vi "CH_LM Config Statistics Histogram Bin Count.vi"(0 "Meter Index":i32, 2 "Number of Bins (7)":i32=7, 5 "error in (no error)":errorcluster, 7 "Timeout / ms (3000)":i32=3000, 8 "Action (query)":bool, 9 "Lock Timeout / ms (1000)":i32=1000) -> (11 "Lock timed out":bool, 14 "Meter Index":i32, 16 "Number of Bins":i32, 19 "error out":errorcluster)   [LabVIEW 2012, in "CH_LM.lvlib"]
doc: "This command will set/query the statistics histogram bin count, which takes effect at the end of the current statistical batch."
uses:
  CH_LM.lvlib
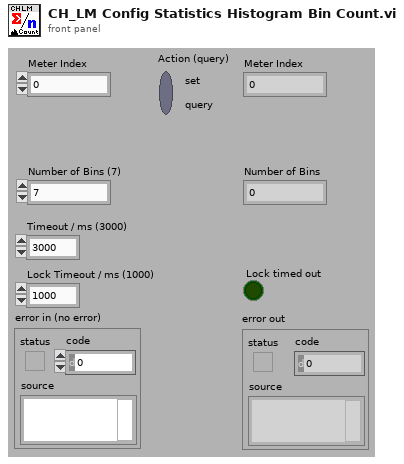
[diagram p1: front panel]
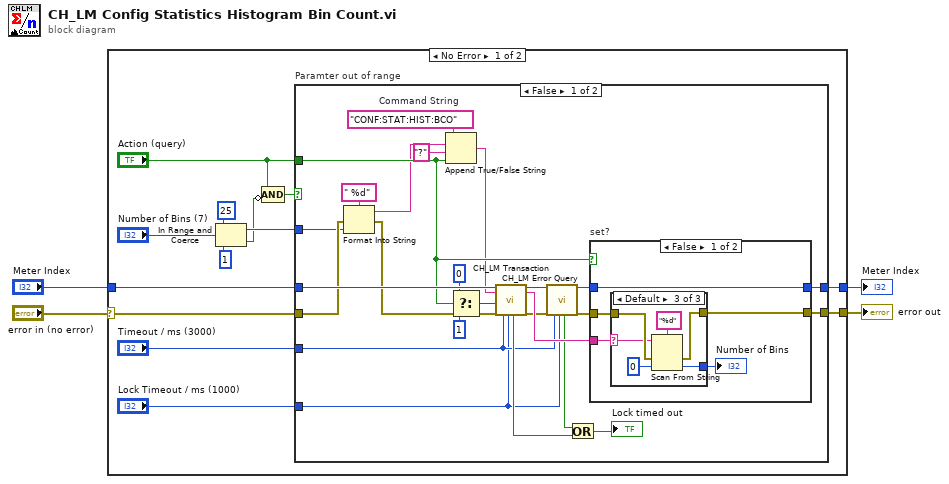
[diagram p0: block diagram]
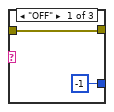
[diagram p2: hidden frame]
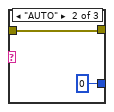
[diagram p3: hidden frame]
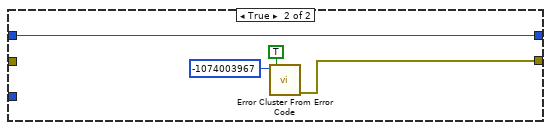
[diagram p5: hidden frame]
diagram:
  n1 = case shown="No Error" "error in (no error)" {
    selector: "error in (no error)" -> [w17 w65]
    tunnel: [w15 w65] -> w4
    tunnel: "Meter Index" -> [w16 w64]
    tunnel: [w14 w64] -> w1
    frame No Error {
      n2 = In Range and Coerce(upper limit=25, x="Number of Bins (7)", lower limit=1) -> (coerced(x)=w11:i32, In Range?=w5:bool)
      n3 = Compound Arithmetic op=AND("Action (query)", invert w5) -> (w7:bool)
      n4 = case "Paramter out of range" shown="False" w7 {
        tunnel: w17 -> [w23 _]
        tunnel: w16 -> [w42 w63]
        tunnel: [w39 w61] -> w15
        tunnel: [w34 w63] -> w14
        tunnel: "Timeout / ms (3000)" -> [w26 _]
        tunnel: "Lock Timeout / ms (1000)" -> [w25 _]
        tunnel: w11 -> [w19 _]
        tunnel: "Action (query)" -> [w24 _]
        frame False {
          w41 = "CONF:STAT:HIST:BCO"  # Command String
          n5 = Format Into String(format string=" %d", error in=w23, w19) -> (resulting string=w20:string, error out=w22:errorcluster)  [unwired: 1 in]
          n6 = Append True/False String(1:w24, 2:"?" ("true string"), 3:w20, 4:w41) -> (0:w21:string)
          n7 = Select(t=0, s=w24, f=1 ("NofStrings (-1:all)")) -> (s? t:f=w36:i32)
          n8 = call "CH_LM Transaction.vi"("Meter Index"=w42, "Command String"=w21, "NofStrings (-1:all)"=w36, "error in (no error)"=w22, "Timeout / ms (3000)"=w26, "Lock Timeout / ms (1000)"=w25) -> ("Lock timed out"=w28:bool, "Meter Index"=w33:i32, "Response"=w40:string, "error out"=w31:errorcluster)  [unwired: 10 out]
          n9 = call "CH_LM Error Query.vi"("Meter Index"=w33, "error in (no error)"=w31, "Timeout / ms (3000)"=w26, "Lock Timeout / ms (1000)"=w25) -> ("Lock timed out"=w29:bool, "Meter Index"=w32:i32, "error out"=w30:errorcluster)  [unwired: 13 out]
          n10 = Or(x=w29, y=w28) -> (x .or. y?=→"Lock timed out":bool)
          n11 = case "set?" shown="False" w24 {
            tunnel: w40 -> [w43 _]
            tunnel: w30 -> [w47 w59]
            tunnel: [w46 w59] -> w39
            tunnel: w32 -> [w45 w58]
            tunnel: [w45 w58] -> w34
            frame False {
              n12 = case shown="Default" w43 {
                selector: w43 -> [_ _ w52]
                tunnel: w47 -> [w48 w51 w57]
                tunnel: [w48 w51 w56] -> w46
                tunnel: [-1 ("default value 1") 0 ("default value 1") w53] -> w44
                frame "OFF" {
                }
                frame "AUTO" {
                }
                frame Default {
                  n13 = Scan From String(format string="%d", input string=w52, error in=w57, default 1=0 ("default value 1")) -> (error out=w56:errorcluster, output 1=w53:i32)  [unwired: 1 in, 2 out]
                }
              }
              "Number of Bins" <- w44
            }
            frame True {
            }
          }
        }
        frame True {
          n14 = call <vilib>:"Error Cluster From Error Code.vi"("show call chain? (False)"=TRUE, "error code (0)"=-1074003967) -> ("error out"=w61:errorcluster)  [unwired: 1 in, 6 out]
        }
      }
    }
    frame Error {
    }
  }
  "error out" <- w4
  "Meter Index" <- w1
